vi "Set IPS PSU Target.vi"(6 "Axis":T1, 8 "error in (no error)":errorcluster, 9 "Target Field Rate (T/min)":dbl format="%#.2f", 10 "Target Field (T)":dbl format="%#.2f", 11 "Instrument.OxfordVRM in":refnum<class "Instrument.OxfordVRM.lvclass">) -> (0 "error out":errorcluster, 2 "Response":string, 3 "Instrument.OxfordVRM out":refnum<class "Instrument.OxfordVRM.lvclass">)   [LabVIEW 2016, in "Instrument.OxfordVRM.lvclass"]
uses:
  Instrument.OxfordVRM.lvclass
  <userlib>/LevyLab/Levylab Instruments/Instrument Types/Cryostat/Typedefs/Magnet Axis--Enum.ctl
  Instrument.OxfordVRM.lvclass/Instrument.OxfordVRM.ctl
  <instrlib>/Mercury iXX/Public/Libraries/Magnet/Open/Open Magnet Device.vi
  <instrlib>/Mercury iXX/Public/Libraries/Magnet/Signals/Set/Target Field Rate (Set).vi
  <instrlib>/Mercury iXX/Public/Libraries/Magnet/Signals/Set/Target Field (Set).vi
  <instrlib>/Mercury iXX/Public/Libraries/Magnet/Signals/Read/Target Field Rate (Read).vi
  <instrlib>/Mercury iXX/Public/Libraries/Magnet/Signals/Read/Target Field (Read).vi
  <instrlib>/Mercury iXX/Mercury iXX.lvlib
  <instrlib>/Mercury iXX/Public/Libraries/Magnet.lvlib
  <userlib>/LevyLab/Levylab Instruments/Instrument Types/Cryostat/Instrument.Cryostat.lvclass
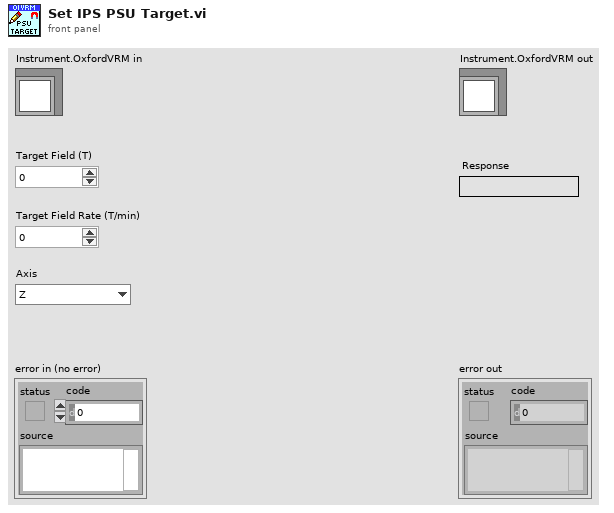
[diagram p1: front panel]
types:
  T1 = typedef "Instrument.Cryostat.lvclass/Magnet Axis--Enum.ctl" = enum16{"Z", "X", "Y"}
  T2 = typedef "Mercury iXX.lvlib/Mercury Reference.ctl" = cluster{"Comms":refnum<visa-resource-name>, "Device ID":string[], "Comms Layer":T3, "Command":string, "Query reference":T4}
  T3 = typedef "Mercury iXX.lvlib/Comms Transport Layer.ctl" = enum16{"Ethernet TCP/IP", "USB", "ISOBus - RS-232", "GPIB"}
  T4 = typedef "Mercury iXX.lvlib/Query Dynamic Reference.ctl" = refnum<vi>
  T5 = typedef "Mercury iXX.lvlib/Response String.ctl" = string
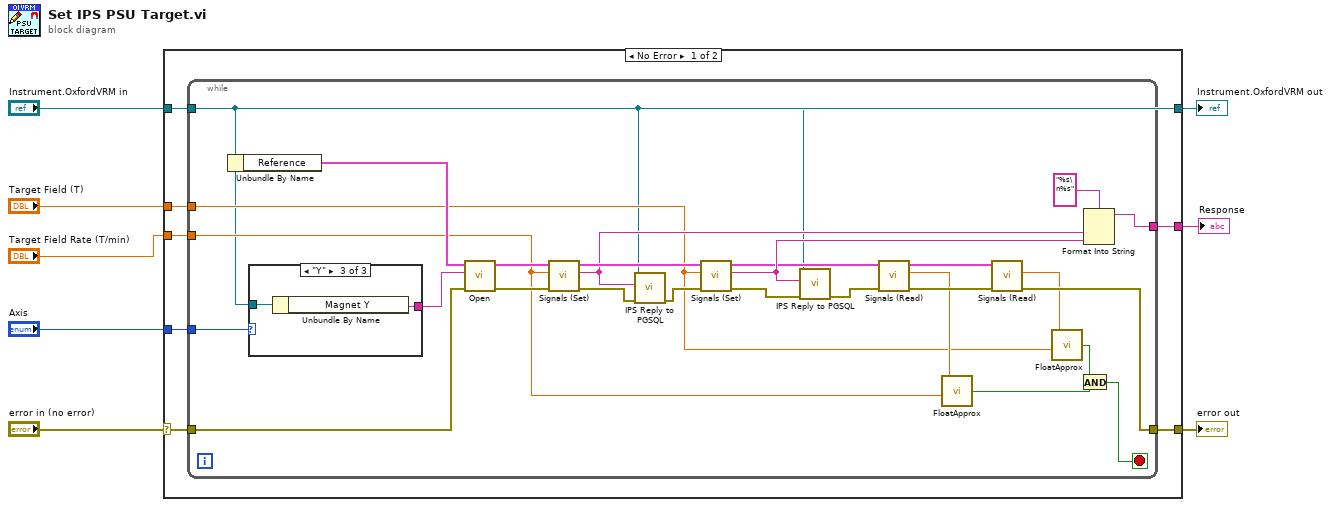
[diagram p0: block diagram]
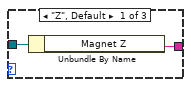
[diagram p2: hidden frame]
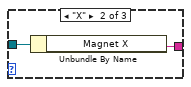
[diagram p3: hidden frame]
diagram:
  n1 = case shown="No Error" "error in (no error)" {
    selector: "error in (no error)" -> [w14 w50]
    tunnel: [w10 w50] -> w7
    tunnel: [w15 w49] -> w5
    tunnel: "Instrument.OxfordVRM in" -> [w15 w49]
    tunnel: [w11 _] -> w4
    tunnel: "Target Field (T)" -> [w13 _]
    tunnel: "Target Field Rate (T/min)" -> [w12 _]
    tunnel: "Axis" -> [w9 _]
    frame No Error {
      n2 = while {
        tunnel: w15 -> [w17]
        tunnel: w14 -> [w41]
        tunnel: w13 -> [w19]
        tunnel: w12 -> [w20]
        tunnel: [w31] -> w11
        tunnel: [w26] -> w10
        tunnel: w9 -> [w18]
        stop <- w21 stop-if-true
        n3 = Unbundle By Name(w17) -> ("Reference"=w42:T2)
        n4 = case shown="\"Y\"" w18 {
          tunnel: [w44 w46 w47] -> w16
          tunnel: w17 -> [w43 w45 w48]
          frame "Z", Default {
            n5 = Unbundle By Name(w43) -> ("Magnet Z"=w44:string)
          }
          frame "X" {
            n6 = Unbundle By Name(w45) -> ("Magnet X"=w46:string)
          }
          frame "Y" {
            n7 = Unbundle By Name(w48) -> ("Magnet Y"=w47:string)
          }
        }
        n8 = call-poly <instrlib>:"Open.vi"("error in (no error)"=w41, "Device Identifier"=w16, "Mercury Reference In"=w42) -> ("error out"=w35:errorcluster, "Mercury Reference Out"=w36:T2)  [unwired: 7 out]
        n9 = call-poly <instrlib>:"Signals (Set).vi"("error in"=w35, "Target Field Rate"=w20, "Mercury Reference In"=w36) -> ("error out"=w39:errorcluster, "Response"=w32:T5, "Mercury Reference Out"=w37:T2)  [unwired: 2 in, 4 out]
        n10 = call "IPS Reply to PGSQL.vi"("error in (no error)"=w39, "Response"=w32, "Instrument.1820 in"=w17) -> ("error out"=w38:errorcluster)  [unwired: 7 in, 1 out]
        n11 = call-poly <instrlib>:"Signals (Set).vi"("error in"=w38, "Target Field"=w19, "Mercury Reference In"=w37) -> ("error out"=w40:errorcluster, "Response"=w33:T5, "Mercury Reference Out"=w29:T2)  [unwired: 2 in, 4 out]
        n12 = call "IPS Reply to PGSQL.vi"("error in (no error)"=w40, "Response"=w33, "Instrument.1820 in"=w17) -> ("error out"=w30:errorcluster)  [unwired: 7 in, 1 out]
        n13 = call-poly <instrlib>:"Signals (Read).vi"("error in"=w30, "Mercury Reference In"=w29) -> ("error out"=w27:errorcluster, "Target Field Rate"=w25:dbl, "Mercury Reference Out"=w28:T2)  [unwired: 5 in, 2 out]
        n14 = call "FloatApprox.vi"("y"=w20, "x"=w25) -> ("x ~ y?"=w22:bool)  [unwired: 4 in]
        n15 = call-poly <instrlib>:"Signals (Read).vi"("error in"=w27, "Mercury Reference In"=w28) -> ("error out"=w26:errorcluster, "Target Field"=w24:dbl)  [unwired: 5 in, 3 out]
        n16 = call "FloatApprox.vi"("y"=w19, "x"=w24) -> ("x ~ y?"=w23:bool)  [unwired: 4 in]
        n17 = And(x=w23, y=w22) -> (x .and. y?=w21:bool)
        n18 = Format Into String(format string="%s\n%s", w32, w33) -> (resulting string=w31:string)  [unwired: 2 in, 1 out]
      }
    }
    frame Error {
    }
  }
  "error out" <- w7
  "Instrument.OxfordVRM out" <- w5
  "Response" <- w4
